vi "png_file_to_image_array.vi"(8 "error in (no error)":errorcluster, 9 "dimension size 2":i32=1920, 10 "dimension size 1":i32=1080, 11 "path to PNG file":path) -> (3 "output array":u8[][](array[numeric]))   [LabVIEW 2025]
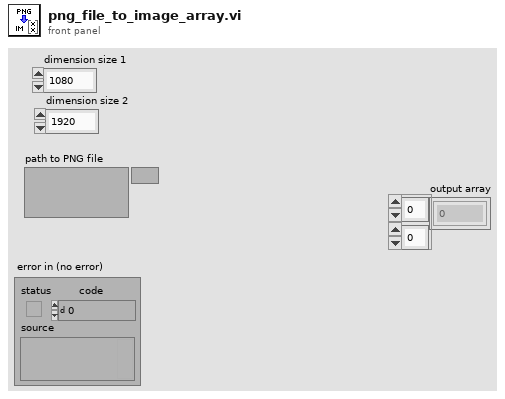
[diagram p1: front panel]
types:
  T1 = typedef "imagedata.ctl" = cluster{"image type":i32, "image depth":i32, "image":u8[], "mask":u8[], "colors":u32[], "Rectangle":cluster{"left":i16, "top":i16, "right":i16, "bottom":i16}}
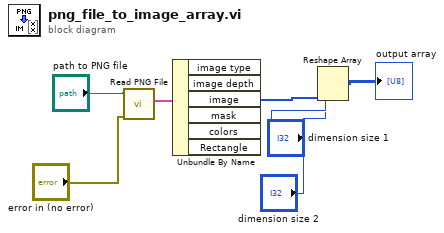
[diagram p0: block diagram]
diagram:
  n1 = call <vilib>:"Read PNG File.vi"("error in (no error)"="error in (no error)", "path to PNG file"="path to PNG file") -> ("image data"=w7:T1)  [unwired: 7 in, 2 out]
  n2 = Unbundle By Name(w7) -> ("image"=w6:u8[])  [unwired: 5 out]
  n3 = Reshape Array(w6, "dimension size 1", "dimension size 2") -> (→"output array":u8[][])
